vi "Open VI Ref at Path Value.vi"(8 "error in (no error)":errorcluster, 11 "VI Reference Control in":refnum<class "VI Reference Control.lvclass">) -> (0 "error out":errorcluster, 3 "VI Reference Control out":refnum<class "VI Reference Control.lvclass">)   [LabVIEW 2016, in "VI Reference Control.lvclass"]
uses:
  VI Reference Control.lvclass
  VI Reference Control.lvclass/VI Reference Control.ctl
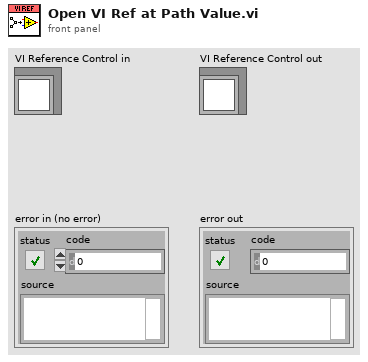
[diagram p1: front panel]
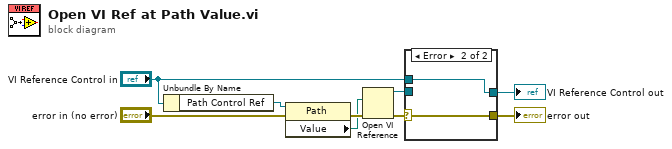
[diagram p0: block diagram]
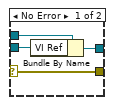
[diagram p2: hidden frame]
diagram:
  n1 = Unbundle By Name("VI Reference Control in") -> ("Path Control Ref"=w6:refnum<vi>)
  n2 = property on="Property Node" class="Path"(reference=w6, error in="error in (no error)") -> (error out=w5:errorcluster, "Value"=w4:path)  [unwired: 1 out]
  n3 = Open VI Reference(vi path=w4, error in (no error)=w5) -> (vi reference=w8:refnum<vi>, error out=w2:errorcluster)  [unwired: 4 in]
  n4 = case shown="Error" w2 {
    selector: w2 -> [w10 w15]
    tunnel: [w13 w14] -> w9
    tunnel: w8 -> [w12 _]
    tunnel: "VI Reference Control in" -> [w11 w14]
    tunnel: [w10 w15] -> w1
    frame No Error {
      n5 = Bundle By Name(cluster=w11, "VI Ref"=w12) -> (w13:refnum<class "VI Reference Control.lvclass">)
    }
    frame Error {
    }
  }
  "error out" <- w1
  "VI Reference Control out" <- w9
